vi "Configure Trigger Source.vi"(8 "error in":errorcluster, 9 "Type":u16(ring) items=["Bus", "Manual"], 11 "VISA resource name":refnum<visa-resource-name>) -> (0 "error out":errorcluster, 3 "VISA resource name out":refnum<visa-resource-name>)   [LabVIEW 2015, in "IT6700H.lvlib"]
doc: "This command is used to select the source of the trigger signal. The power supply can receive a Trigger signal from the panel (keyboard trigger key) or a bus trigger signal. When the *RST command is executed, the trigger source is set to MANUAL.\n<b>Type</b>\n0: Bus\n1: Manual"
uses:
  <instrlib>/IT6700H/IT6700H.lvlib
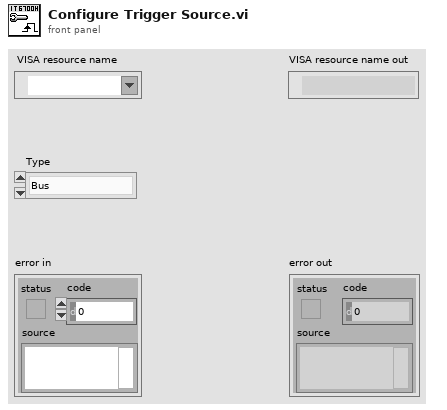
[diagram p1: front panel]
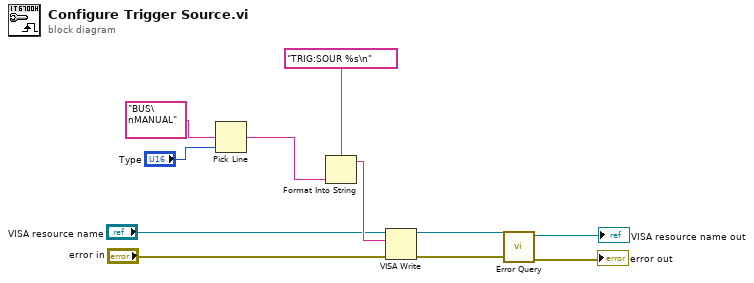
[diagram p0: block diagram]
diagram:
  n1 = Pick Line(multi-line string="BUS\nMANUAL", line index="Type") -> (output string=w9:string)  [unwired: 1 in]
  n2 = Format Into String(format string="TRIG:SOUR %s\n", w9) -> (resulting string=w7:string)  [unwired: 2 in, 1 out]
  n3 = VISA Write(VISA resource name="VISA resource name", write buffer=w7, error in (no error)="error in") -> (VISA resource name out=w4:refnum<visa-resource-name>, error out=w3:errorcluster)  [unwired: 1 out]
  n4 = call <instrlib>:"Error Query.vi"("error in"=w3, "VISA resource name"=w4) -> ("error out"=→"error out":errorcluster, "VISA resource name out"=→"VISA resource name out":refnum<visa-resource-name>)  [unwired: 6 in, 2 out]
